vi "scaleParameter.set.vi"(8 "error in (no error)":errorcluster, 10 "scaleParameter":refnum<class "scaleParameter.lvclass">, 11 "noManifest in":refnum<class "noManifest.lvclass">) -> (0 "error out":errorcluster, 3 "noManifest out":refnum<class "noManifest.lvclass">)   [LabVIEW 2020, in "nominal types.lvlib" / "timestampManifest.lvlib" / "noManifest.lvclass"]
uses:
  noManifest.lvclass
  scaleParameter/scaleParameter.lvclass
  noManifest.lvclass/noManifest.ctl
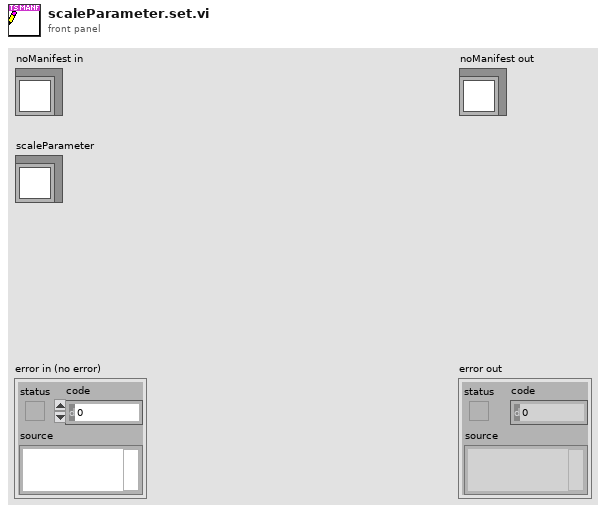
[diagram p1: front panel]
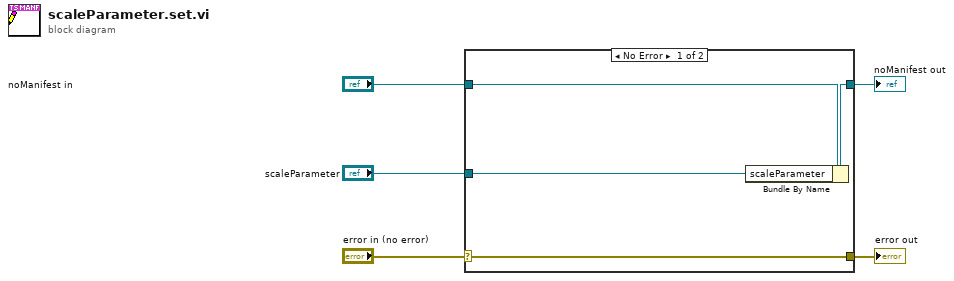
[diagram p0: block diagram]
diagram:
  n1 = case shown="No Error" "error in (no error)" {
    selector: "error in (no error)" -> [w9 w10]
    tunnel: [w9 w10] -> w4
    tunnel: [w7 w11] -> w2
    tunnel: "noManifest in" -> [w8 w11]
    tunnel: "scaleParameter" -> [w6 _]
    frame No Error {
      n2 = Bundle By Name(cluster=w8, "scaleParameter"=w6) -> (w7:refnum<class "noManifest.lvclass">)
    }
    frame Error {
    }
  }
  "error out" <- w4
  "noManifest out" <- w2
